vi "Configure.vi"(8 "error in (no error)":errorcluster, 11 "AOTF in":refnum<class "Invivo_AOTF.lvclass">) -> (0 "error out":errorcluster, 2 "cancelled?":bool, 3 "AOTF out":refnum<class "Invivo_AOTF.lvclass">)   [LabVIEW 2012, in "Invivo_AOTF.lvclass"]
doc: "The configure method configures the details for the RabbitMQ connection. \n\nIn the derived class, make a call to the parent for setting these parameters."
uses:
  Invivo_AOTF.lvclass
  <vilib>/Utility/miscctls.llb/LVPointTypeDef.ctl
  Invivo_AOTF.lvclass/Invivo_AOTF.ctl
  <vilib>/Distrio/Murmex/Murmex/Murmex.lvclass
panel:
  in  "Tab Control":enum32{"Comport", "Debug"}(tab)
  in  "VISA Wait":dbl[unit]=0.2
  in  "Power LUT file":path=path "C:/DATA/Programming/Giorgio/AOTF-InVivoSPIM/AOTF.txt"
  in  "Baud rate":u32=19200
  in  "button::configure murmex":bool
  in  "button::ok":bool
  in  "button::cancel":bool
  in  "VISA resource name":refnum<visa-resource-name>="COM1"
  in  "Time out":u32=2000
  # "RabbitMQ parameters"
  # "Window position"
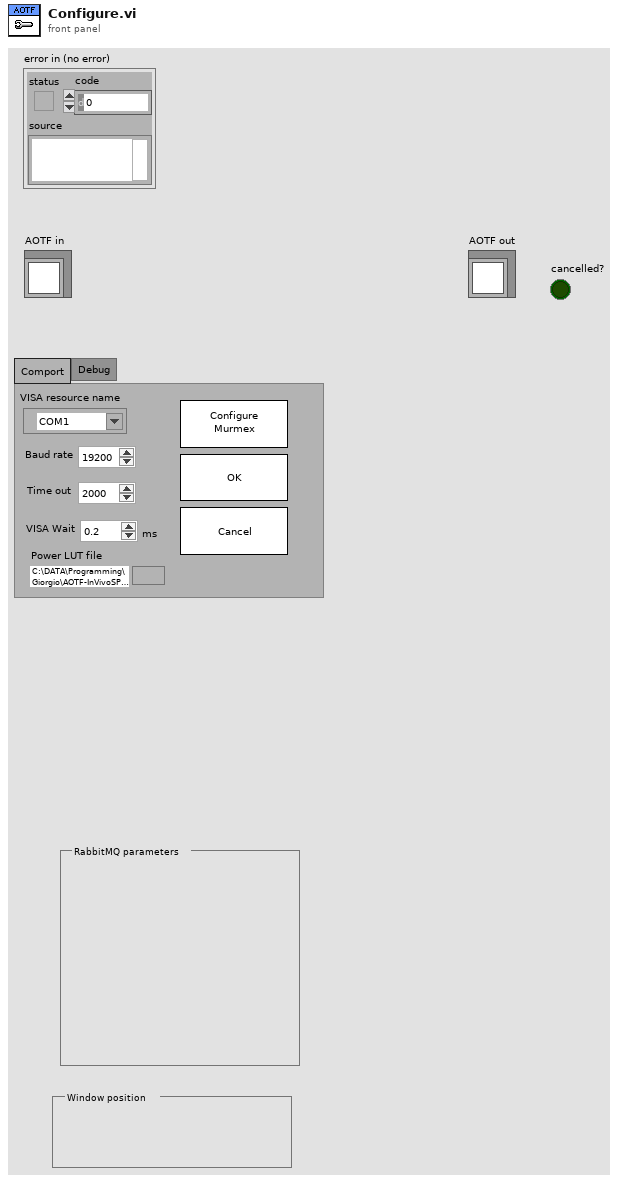
[diagram p1: front panel]
types:
  T1 = typedef "LVPointTypeDef.ctl" = cluster{"Horizontal":i16, "Vertical":i16}
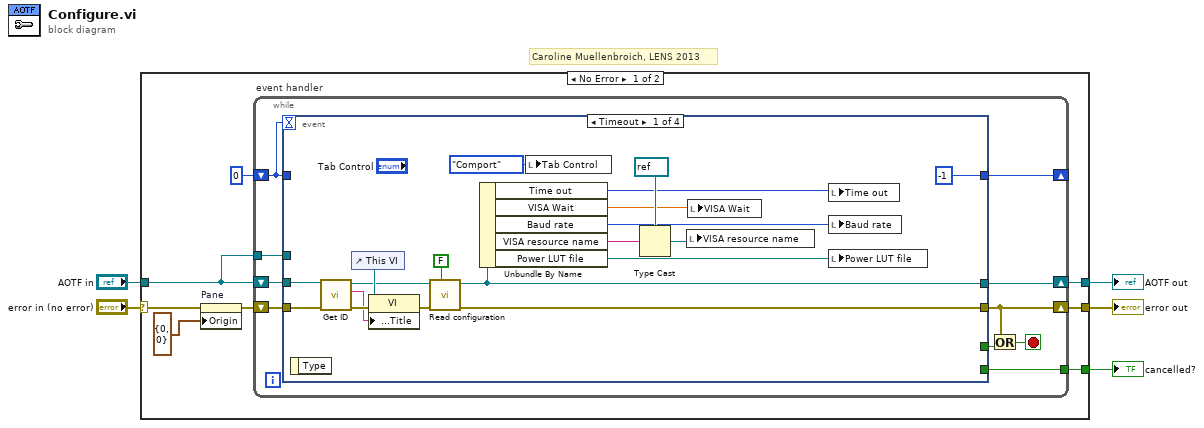
[diagram p0: block diagram]
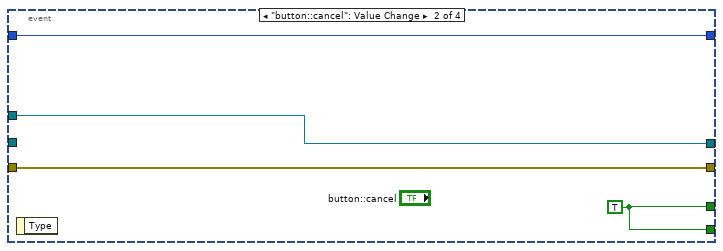
[diagram p2: hidden frame]
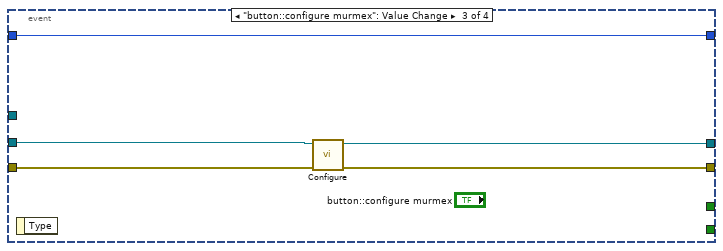
[diagram p3: hidden frame]
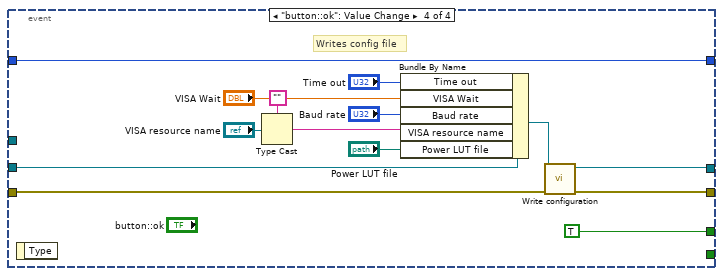
[diagram p4: hidden frame]
diagram:
  # "Caroline Muellenbroich, LENS 2013"
  n1 = case shown="No Error" "error in (no error)" {
    selector: "error in (no error)" -> [w11 w66]
    tunnel: "AOTF in" -> [w12 w67]
    tunnel: [w8 w66] -> w1
    tunnel: [w7 w67] -> w3
    tunnel: [w6 _] -> w2
    frame No Error {
      n2 = property on="Pane" class="Pane"(error in=w11, "Origin"=T1 {"Horizontal"=0, "Vertical"=0}) -> (error out=w10:errorcluster)  [unwired: 1 in, 1 out]
      n3 = while "event handler" {
        shift-right: [w23] -> _
        shift-left: 0 -> [w14]
        shift-right: [w19] -> w7
        shift-left: w12 -> [w22]
        tunnel: w12 -> [w21]
        shift-right: [w17] -> w8
        shift-left: w10 -> [w20]
        tunnel: [w15] -> w6
        stop <- w18 stop-if-true
        n4 = event shown="[0] Timeout" {
          selector: _ -> [_ _ _ _]
          dyn-events: _ -> [_ _ _ _]
          timeout: w14 -> [_ _ _ _]
          tunnel: w14 -> [_ w46 w51 w65]
          tunnel: [-1 w46 w51 w65] -> w23
          tunnel: w22 -> [w38 _ w48 w62]
          tunnel: w21 -> [_ w43 _ _]
          tunnel: w20 -> [w41 w44 w47 w57]
          tunnel: [w33 w43 w49 w63] -> w19
          tunnel: [w32 w44 w50 w64] -> w17
          tunnel: [_ w45 _ TRUE ("force loading?")] -> w16
          tunnel: [_ w45 _ _] -> w15
          event Timeout {
            n5 = event-data() -> ()  [unwired: 1 in, 1 out]
            n6 = call <vilib>:"Get ID.vi"("error in (no error)"=w41, "Murmex in"=w38) -> ("error out"=w39:errorcluster, "component id"=w37:string, "Murmex out"=w35:refnum<class "Invivo_AOTF.lvclass">)  [unwired: 7 in]
            n7 = control-ref of="This VI"() -> (w40:refnum<vi>)
            n8 = property class="VI"(reference=w40, error in=w39, "Front Panel.Title"=w37) -> (error out=w36:errorcluster)  [unwired: 1 out]
            n9 = call-dynamic "Read configuration.vi"("force loading?"=FALSE, "error in (no error)"=w36, "AOTF in"=w35) -> ("error out"=w32:errorcluster, "AOTF out"=w33:refnum<class "Invivo_AOTF.lvclass">)  [unwired: 7 in]
            n10 = Unbundle By Name(w33) -> ("Time out"=w27:u32, "VISA Wait"=w24:dbl[unit], "Baud rate"=w26:u32, "VISA resource name"=w30:string, "Power LUT file"=w25:path)
            n11 = local write "Tab Control"(enum32{"Comport", "Debug"}."Comport" ("Tab Control")) -> ()
            n12 = Type Cast(type=refnum<visa-resource-name> refnum ("VISA resource name"), x=w30) -> (*(type *) &x=w29:refnum<visa-resource-name>)
            n13 = local write "VISA resource name"(w29) -> ()
            n14 = local write "VISA Wait"(w24) -> ()
            n15 = local write "Time out"(w27) -> ()
            n16 = local write "Baud rate"(w26) -> ()
            n17 = local write "Power LUT file"(w25) -> ()
          }
          event "button::cancel": Value Change {
            w45 = TRUE ("force loading?")
            n18 = event-data() -> ()  [unwired: 1 in, 1 out]
          }
          event "button::configure murmex": Value Change {
            n19 = event-data() -> ()  [unwired: 1 in, 1 out]
            n20 = call-parent "Configure.vi"("error in (no error)"=w47, "Murmex in"=w48) -> ("error out"=w50:errorcluster, "Murmex out"=w49:refnum<class "Invivo_AOTF.lvclass">)  [unwired: 7 in, 1 out]
          }
          event "button::ok": Value Change {
            # "Writes config file"
            n21 = event-data() -> ()  [unwired: 1 in, 1 out]
            n22 = Type Cast(type="", x="VISA resource name") -> (*(type *) &x=w59:string)
            n23 = Bundle By Name(cluster=w62, "Time out"="Time out", "VISA Wait"="VISA Wait", "Baud rate"="Baud rate", "VISA resource name"=w59, "Power LUT file"="Power LUT file") -> (w61:refnum<class "Invivo_AOTF.lvclass">)
            n24 = call-dynamic "Write configuration.vi"("error in (no error)"=w57, "AOTF in"=w61) -> ("error out"=w64:errorcluster, "AOTF out"=w63:refnum<class "Invivo_AOTF.lvclass">)  [unwired: 8 in]
          }
        }
        n25 = Or(x=w17, y=w16) -> (x .or. y?=w18:bool)
      }
    }
    frame Error {
    }
  }
  "error out" <- w1
  "AOTF out" <- w3
  "cancelled?" <- w2
